vi "GT Get Compensate2D Table.vi"(7 "pExternComp":i16, 8 "error in (no error)":errorcluster caption="错误输入（无错误）", 9 "pTable":T1, 10 "tableIndex":i16, 11 "cardNum":i16) -> (0 "error out":errorcluster caption="错误输出", 1 "pTable out":T1, 3 "function return":i16, 5 "pExternComp out":i16)   [LabVIEW 2020, in "gts.lvlib"]
doc: "GT_API GT_GetCompensate2DTable(short cardNum,short tableIndex,TCompensate2DTable *pTable,short *pExternComp=NULL);"
uses:
  gts.lvlib
  dll/32bit/multi_card/gts.dll
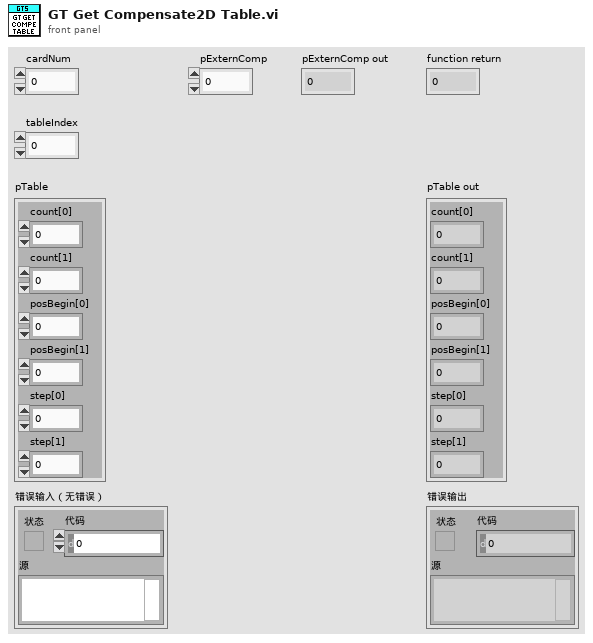
[diagram p1: front panel]
types:
  T1 = cluster{"count[0]":i16, "count[1]":i16, "posBegin[0]":i32, "posBegin[1]":i32, "step[0]":i32, "step[1]":i32}
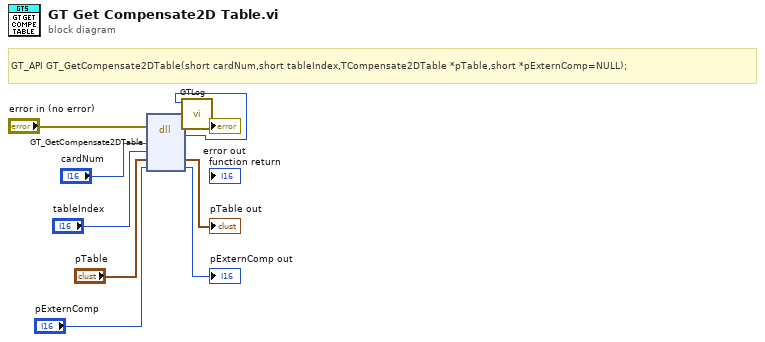
[diagram p0: block diagram]
diagram:
  # "GT_API GT_GetCompensate2DTable(short cardNum,short tableIndex,TCompensate2DTable *pTable,short *pExternComp=NULL);"
  n1 = dll-call lib="C:/1228/dll/32bit/multi_card/gts.dll" fn="GT_GetCompensate2DTable"(error in="error in (no error)", "cardNum"="cardNum", "tableIndex"="tableIndex", "pTable"="pTable", "pExternComp"="pExternComp") -> (error out=w3:errorcluster, w1:i16, "pTable"=→"pTable out":T1, "pExternComp"=→"pExternComp out":i16)  [unwired: 4 in, 1 out]
  n2 = call "GTLog.vi"("error in (no error)"=w3, "Numeric"=w1) -> ("error out"=→"error out":errorcluster)  [unwired: 9 in]
